vi "InCar_timestamp.vi"() -> ()   [LabVIEW 2024]
panel:
  out "producerイベントコード 2":dbl
  out "date/time string":string
  out "producerイベントコード":dbl
  in  "送信":bool
  in  "イベントコード":dbl
  out "Array":dbl[][](array[numeric])
  out "イベントループ":bool
  out "終了フラグ 2":bool
  out "終了フラグ":bool=TRUE
  in  "終了":bool
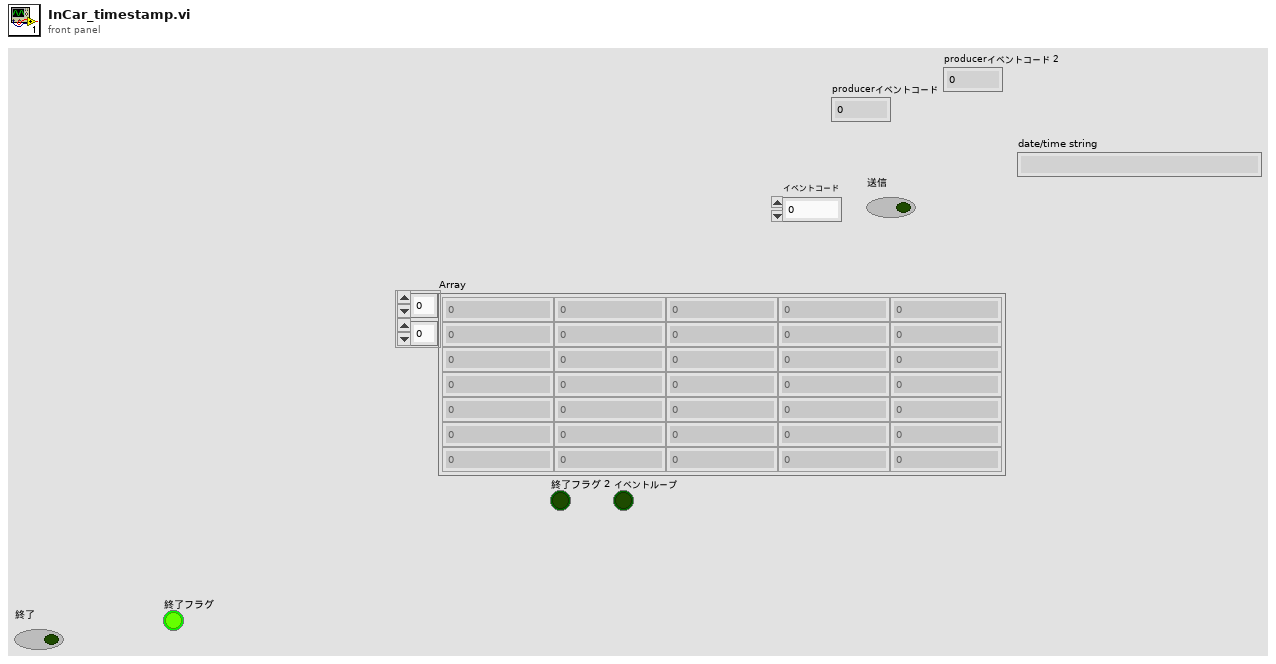
[diagram p1: front panel]
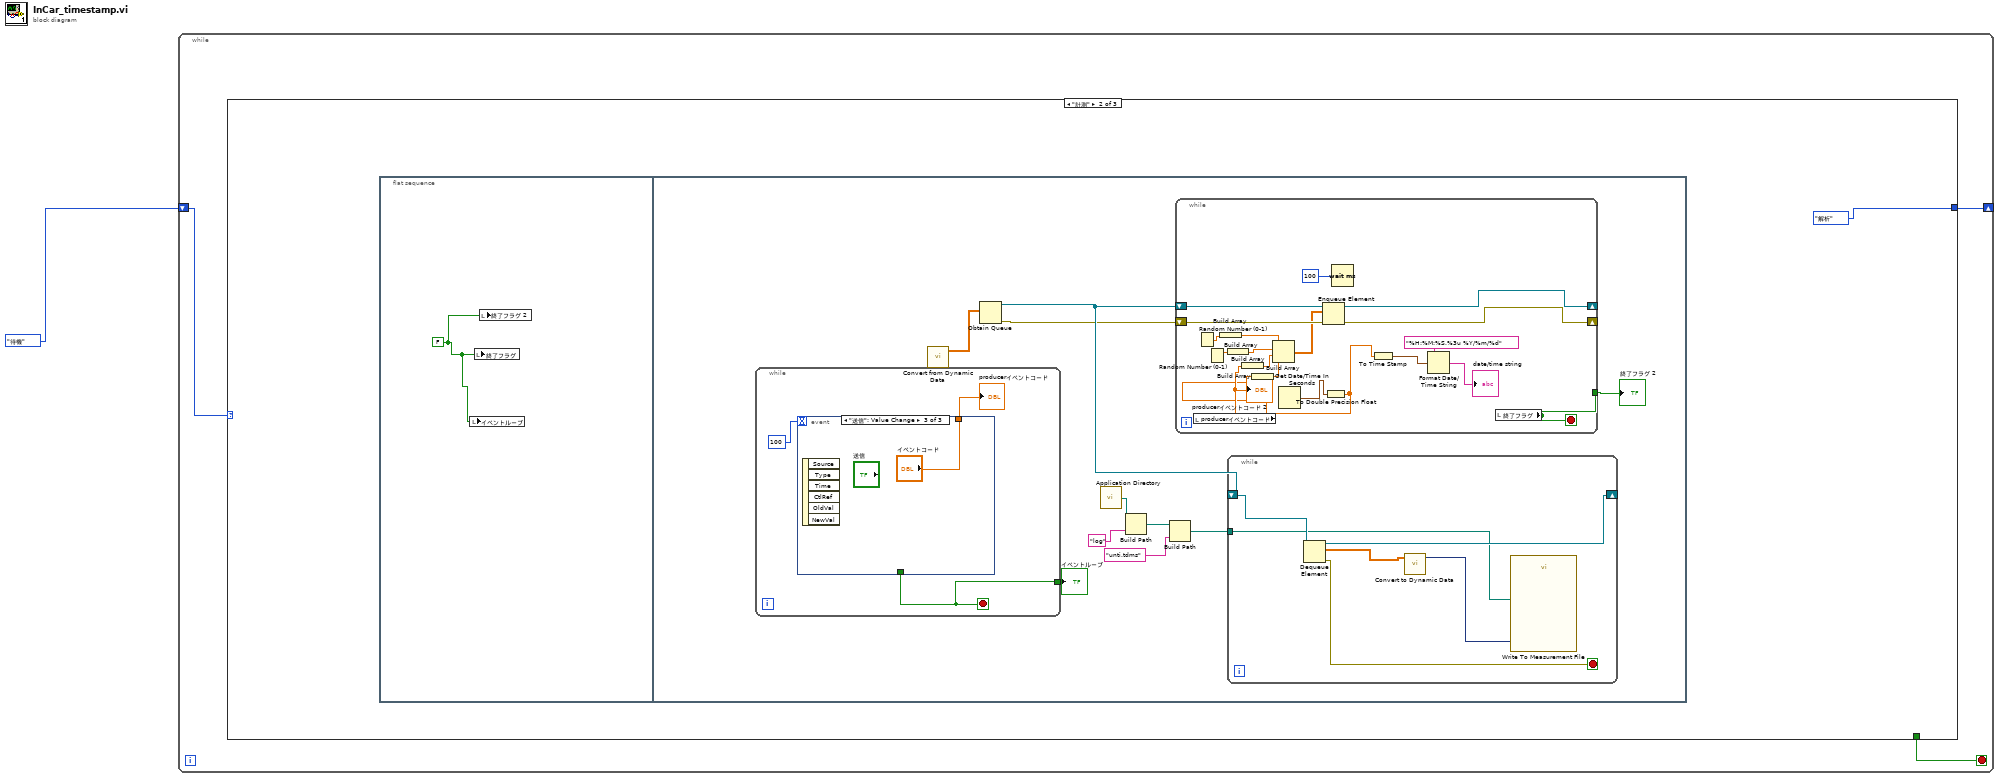
[diagram p0: block diagram]
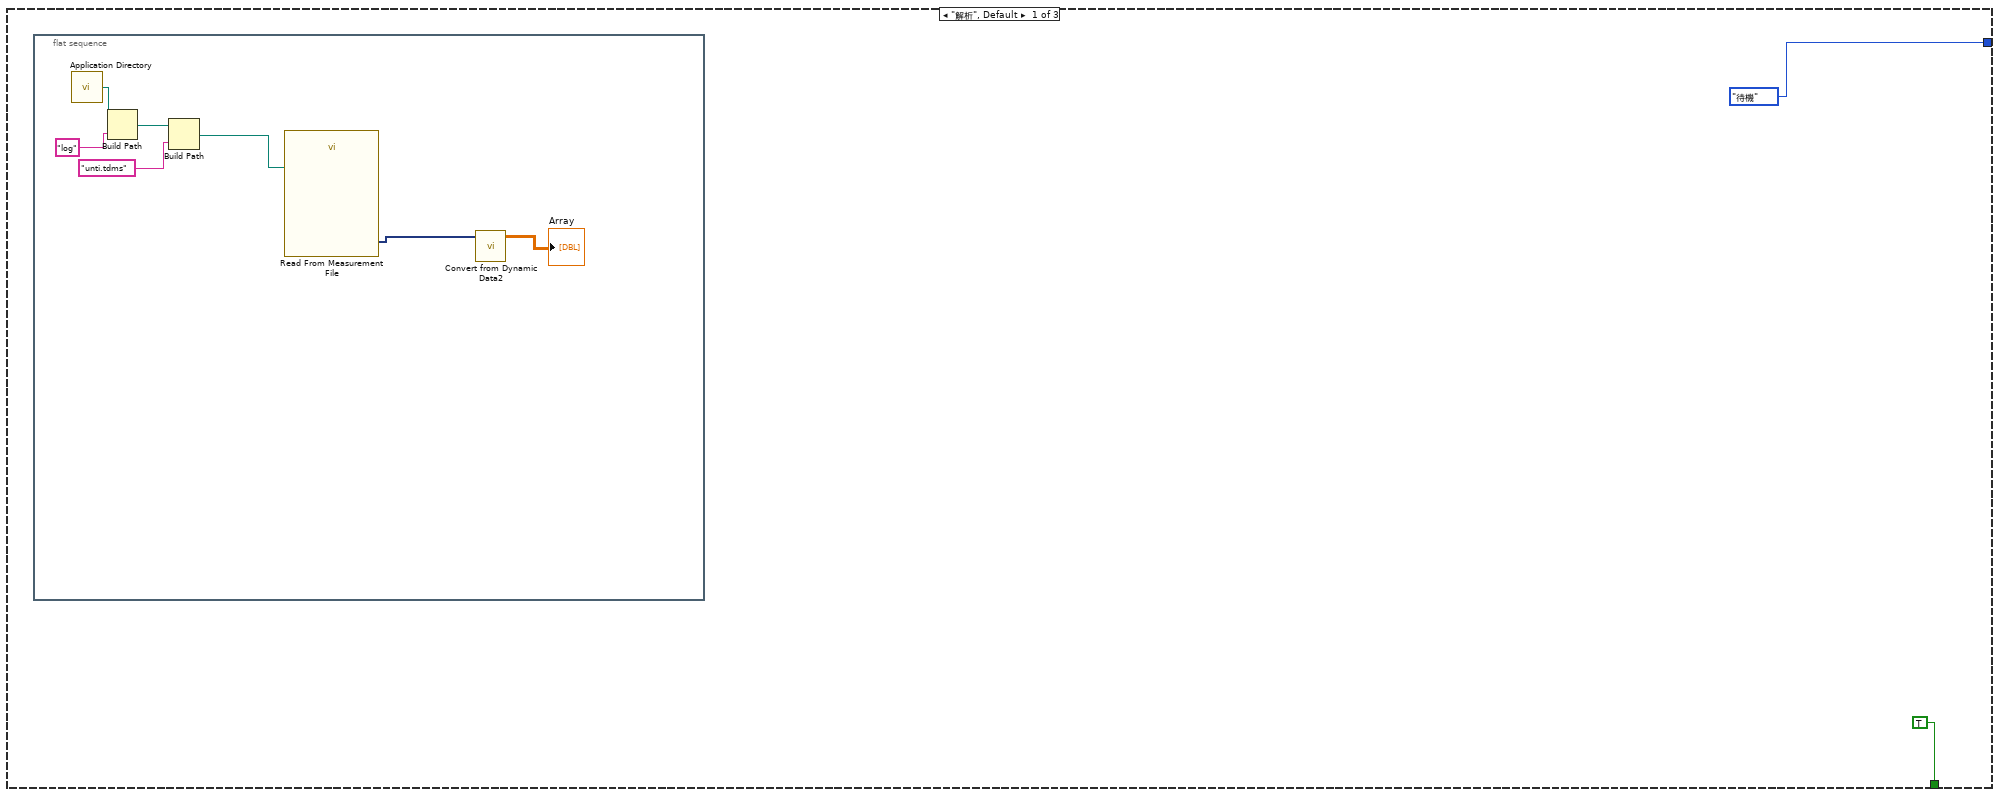
[diagram p2: hidden frame]
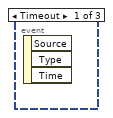
[diagram p3: hidden frame]
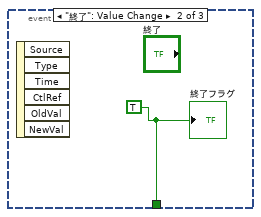
[diagram p4: hidden frame]
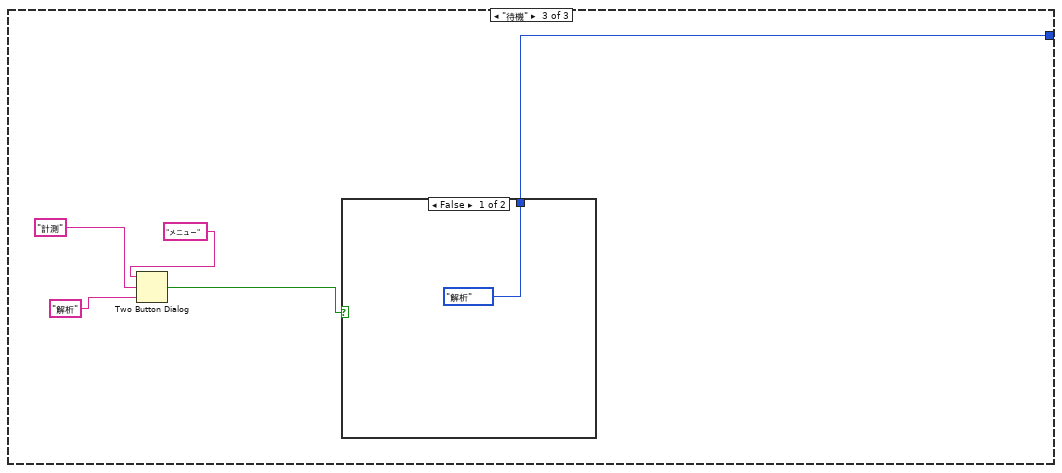
[diagram p5: hidden frame]
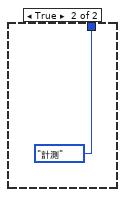
[diagram p6: hidden frame]
diagram:
  n1 = while {
    shift-right: [w3] -> _
    shift-left: enum16{"待機", "解析", "計測"}."待機" -> [w4]
    stop <- w2 stop-if-true
    n2 = case shown="\"計測\"" w4 {
      tunnel: [enum16{"待機", "解析", "計測"}."待機" enum16{"待機", "解析", "計測"}."解析" w57] -> w3
      tunnel: [TRUE _ _] -> w2
      frame "解析", Default {
        n3 = flat-sequence {
          frame #0 {
            n4 = call <vilib>:"Application Directory.vi"() -> ("Application Directory"=w12:path)
            n5 = Build Path(base path=w12, name or relative path="log") -> (appended path=w11:path)
            n6 = Build Path(base path=w11, name or relative path="unti.tdms") -> (appended path=w9:path)
            n7 = call "Read From Measurement File"("Filename"=w9) -> ("Signals"=w8:dynamicdata)  [unwired: 5 in, 5 out]
            n8 = call "Convert from Dynamic Data2"("Dynamic Data Type"=w8) -> ("Array"=→"Array":dbl[][])  [unwired: 3 in]
          }
        }
      }
      frame "計測" {
        n9 = flat-sequence {
          frame #0 {
            w15 = FALSE
            n10 = local write "イベントループ"(w15) -> ()
            n11 = local write "終了フラグ"(w15) -> ()
            n12 = local write "終了フラグ 2"(w15) -> ()
          }
          frame #1 {
            n13 = while {
              tunnel: [w27] -> w21
              stop <- w27 stop-if-true
              n14 = event shown="[2] \"送信\": Value Change" {
                selector: _ -> [_ _ _]
                dyn-events: _ -> [_ _ _]
                timeout: 100 -> [_ _ _]
                tunnel: [_ w29 _] -> w27
                tunnel: [_ _ "イベントコード"] -> w26
                event Timeout {
                  n15 = event-data() -> ()  [unwired: 1 in, 3 out]
                }
                event "終了": Value Change {
                  w29 = TRUE
                  n16 = event-data() -> ()  [unwired: 1 in, 6 out]
                  "終了フラグ" <- w29
                }
                event "送信": Value Change {
                  n17 = event-data() -> ()  [unwired: 1 in, 6 out]
                }
              }
              "producerイベントコード" <- w26
            }
            "イベントループ" <- w21
            n18 = call "Convert from Dynamic Data"() -> ("Array"=w23:dbl[][])  [unwired: 4 in]
            n19 = Obtain Queue(element data type=w23) -> (queue out=w25:refnum<queue>, error out=w24:errorcluster)  [unwired: 4 in, 1 out]
            n20 = call <vilib>:"Application Directory.vi"() -> ("Application Directory"=w19:path)
            n21 = Build Path(base path=w19, name or relative path="log") -> (appended path=w20:path)
            n22 = Build Path(base path=w20, name or relative path="unti.tdms") -> (appended path=w16:path)
            n23 = while {
              shift-right: [w52] -> _
              shift-left: w25 -> [w54]
              shift-right: [w47] -> _
              shift-left: w24 -> [w53]
              tunnel: [w46] -> w22
              stop <- w46 stop-if-true
              n24 = local read "producerイベントコード"() -> (w44:dbl)
              "producerイベントコード 2" <- w44
              n25 = Random Number (0-1)() -> (number: 0 to 1=w49:dbl)
              n26 = Random Number (0-1)() -> (number: 0 to 1=w48:dbl)
              n27 = Build Array(w49) -> (w51:dbl[])
              n28 = Build Array(w48) -> (w50:dbl[])
              n29 = Build Array(w44) -> (w45:dbl[])
              n30 = Get Date/Time In Seconds() -> (seconds since 1Jan1904=w43:timestamp)
              n31 = To Double Precision Float(number=w43) -> (double precision float=w41:dbl)
              n32 = Build Array(w41) -> (w42:dbl[])
              n33 = Build Array(w51, w50, w45, w42) -> (w37:dbl[][])
              n34 = Enqueue Element(queue=w54, element=w37, error in (no error)=w53) -> (queue out=w52:refnum<queue>, error out=w47:errorcluster)  [unwired: 1 in, 1 out]
              n35 = Wait (ms)(milliseconds to wait=100) -> ()  [unwired: 1 out]
              n36 = To Time Stamp(1:w41) -> (0:w40:timestamp)
              n37 = Format Date/Time String(time format string (%c)="%H:%M:%S.%3u %Y/%m/%d", seconds (now)=w40) -> (date/time string=→"date/time string":string)  [unwired: 1 in]
              n38 = local read "終了フラグ"() -> (w46:bool)
            }
            "終了フラグ 2" <- w22
            n39 = while {
              shift-right: [w33] -> _
              shift-left: w25 -> [w36]
              tunnel: w16 -> [w31]
              stop <- w32 stop-if-true
              n40 = Dequeue Element(queue=w36) -> (queue out=w33:refnum<queue>, element=w35:dbl[][], error out=w32:errorcluster)  [unwired: 2 in, 1 out]
              n41 = call "Convert to Dynamic Data"("2D Array"=w35) -> ("Dynamic Data Type"=w34:dynamicdata)  [unwired: 3 in]
              n42 = call "Write To Measurement File"("Signals"=w34, "Filename"=w31) -> ()  [unwired: 15 in, 3 out]
            }
          }
        }
      }
      frame "待機" {
        n43 = Two Button Dialog(message="メニュー", 1:"解析", 2:"計測") -> (T button?=w58:bool)
        n44 = case shown="False" w58 {
          tunnel: [enum16{"待機", "解析", "計測"}."解析" enum16{"待機", "解析", "計測"}."計測"] -> w57
          frame False {
          }
          frame True {
          }
        }
      }
    }
  }
